vi "moveToTargetPosition.vi"(1 "speed":dbl=2000.0 min=0.0 max=2000.0, 2 "Encoder COM Port":refnum<visa-resource-name>, 3 "targetPos":dbl, 4 "currentPos":dbl) -> (0 "updatedCurrentPos":dbl)   [LabVIEW 2013]
panel:
  # "The default motor speed is 2000 steps/second."
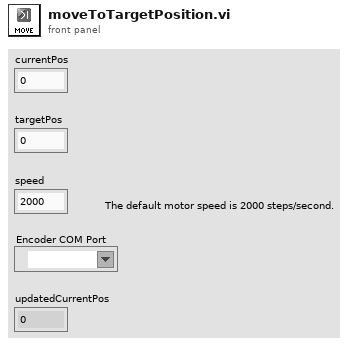
[diagram p1: front panel]
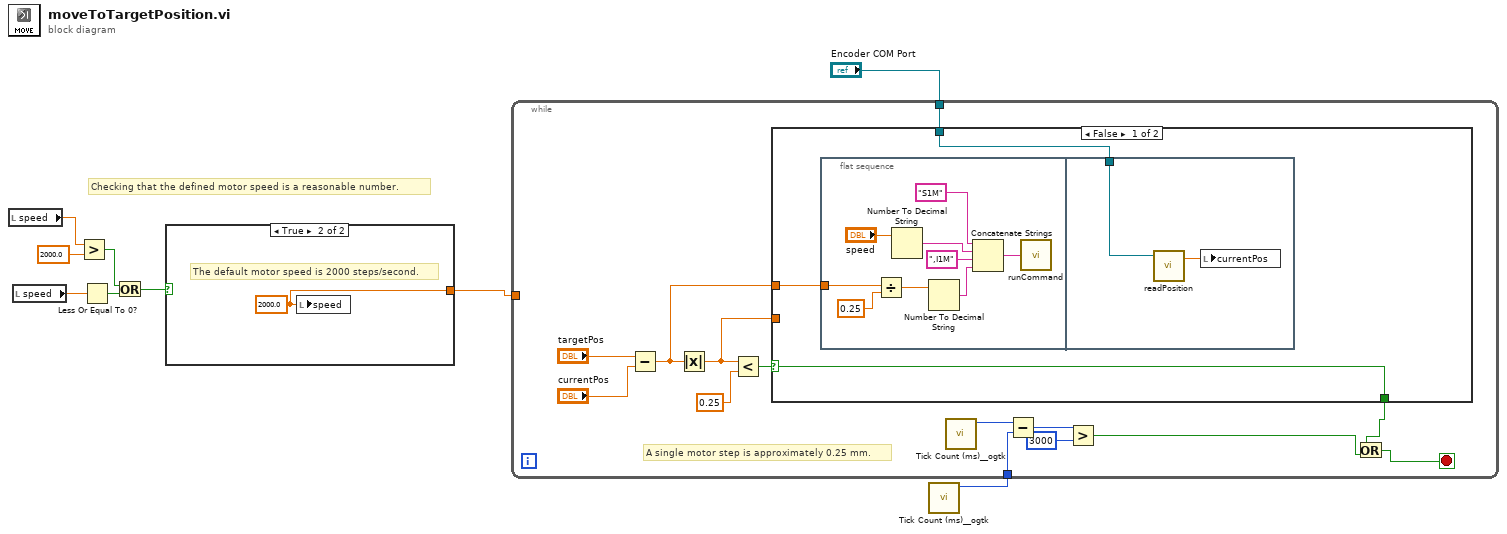
[diagram p0: block diagram]
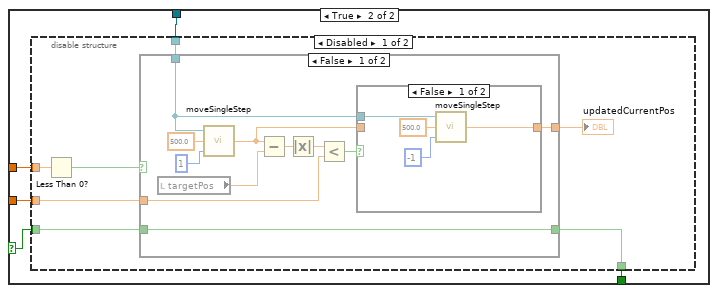
[diagram p3: hidden frame]
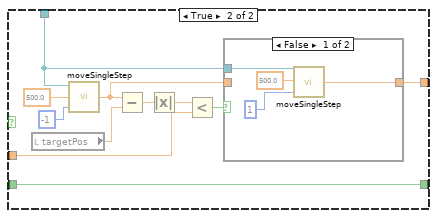
[diagram p5: hidden frame]
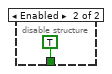
[diagram p7: hidden frame]
diagram:
  # "Checking that the defined motor speed is a reasonable number."
  n1 = local read "speed"() -> (w7:dbl)
  n2 = local read "speed"() -> (w4:dbl)
  n3 = Greater?(x=w7, y=2000.0) -> (0:w8:bool)
  n4 = Less Or Equal To 0?(x=w4) -> (x <= 0?=w6:bool)
  n5 = Or(x=w8, y=w6) -> (x .or. y?=w9:bool)
  n6 = case shown="True" w9 {
    tunnel: [_ w10] -> w2
    frame False {
    }
    frame True {
      w10 = 2000.0 ("speed")
      # "The default motor speed is 2000 steps/second."
      n7 = local write "speed"(w10) -> ()
    }
  }
  n8 = call <userlib>:"Tick Count (ms)__ogtk.vi"() -> ("millisecond timer value"=w1:u32)  [unwired: 10 in, 1 out]
  n9 = while {
    tunnel: "Encoder COM Port" -> [w18]
    tunnel: w2 -> [_]
    tunnel: w1 -> [w16]
    stop <- w11 stop-if-true
    # "A single motor step is approximately 0.25 mm."
    n10 = Subtract(x="targetPos", y="currentPos") -> (x-y=w21:dbl)
    n11 = Absolute Value(x=w21) -> (abs(x)=w19:dbl)
    n12 = Less?(x=w19, y=0.25) -> (x < y?=w22:bool)
    n13 = case shown="False" w22 {
      selector: w22 -> [w26 w41]
      tunnel: w21 -> [w27 w43]
      tunnel: w19 -> [_ w42]
      tunnel: [w26 w40] -> w12
      tunnel: w18 -> [w25 w39]
      frame False {
        n14 = flat-sequence {
          tunnel: w27 -> [w34]
          tunnel: w25 -> [w37]
          frame #0 {
            n15 = Divide(x=w34, y=0.25) -> (x/y=w32:dbl)
            n16 = Number To Decimal String(number="speed") -> (decimal integer string=w29:string)  [unwired: 1 in]
            n17 = Number To Decimal String(number=w32) -> (decimal integer string=w36:string)  [unwired: 1 in]
            n18 = Concatenate Strings("S1M" ("string"), w29, ",I1M" ("string"), w36) -> (w35:string)
            n19 = call "runCommand.vi"("command"=w35) -> ()  [unwired: 1 in]
          }
          frame #1 {
            n20 = call "readPosition.vi"("VISA resource name"=w37) -> ("position"=w38:dbl)  [unwired: 1 in, 2 out]
            n21 = local write "currentPos"(w38) -> ()
          }
        }
      }
      frame True {
        n22 = disable-structure shown="Disabled" {
          disable-tunnel: w43 -> [w50 _]
          disable-tunnel: w42 -> [w48 _]
          disable-tunnel: w41 -> [w47 _]
          disable-tunnel: [w46 TRUE] -> w40
          disable-tunnel: w39 -> [w44 _]
          frame Disabled {
            n23 = Less Than 0?(x=w50) -> (x < 0?=w49:bool)
            n24 = case shown="False" w49 {
              tunnel: w44 -> [w54 w71]
              tunnel: w48 -> [w55 w72]
              tunnel: w47 -> [w52 w68]
              tunnel: [w53 w69] -> w45
              tunnel: [w52 w68] -> w46
              frame False {
                n25 = local read "targetPos"() -> (w57:dbl)
                n26 = call "moveSingleStep.vi"("direction"=1, "motorSpeed"=500.0, "VISA resource name"=w54) -> ("position"=w61:dbl)
                n27 = Subtract(x=w61, y=w57) -> (x-y=w58:dbl)
                n28 = Absolute Value(x=w58) -> (abs(x)=w59:dbl)
                n29 = Less?(x=w59, y=w55) -> (x < y?=w60:bool)
                n30 = case shown="False" w60 {
                  tunnel: w61 -> [_ w66]
                  tunnel: w54 -> [w64 _]
                  tunnel: [w63 w66] -> w53
                  frame False {
                    n31 = call "moveSingleStep.vi"("direction"=-1, "motorSpeed"=500.0, "VISA resource name"=w64) -> ("position"=w63:dbl)
                  }
                  frame True {
                  }
                }
              }
              frame True {
                n32 = local read "targetPos"() -> (w76:dbl)
                n33 = call "moveSingleStep.vi"("direction"=-1, "motorSpeed"=500.0, "VISA resource name"=w71) -> ("position"=w70:dbl)
                n34 = Subtract(x=w70, y=w76) -> (x-y=w75:dbl)
                n35 = Absolute Value(x=w75) -> (abs(x)=w73:dbl)
                n36 = Less?(x=w73, y=w72) -> (x < y?=w74:bool)
                n37 = case shown="False" w74 {
                  tunnel: w71 -> [w81 _]
                  tunnel: w70 -> [_ w82]
                  tunnel: [w79 w82] -> w69
                  frame False {
                    n38 = call "moveSingleStep.vi"("direction"=1, "motorSpeed"=500.0, "VISA resource name"=w81) -> ("position"=w79:dbl)
                  }
                  frame True {
                  }
                }
              }
            }
            "updatedCurrentPos" <- w45
          }
          frame Enabled {
          }
        }
      }
    }
    n39 = call <userlib>:"Tick Count (ms)__ogtk.vi"() -> ("millisecond timer value"=w17:u32)  [unwired: 10 in, 1 out]
    n40 = Subtract(x=w17, y=w16) -> (x-y=w15:u32)
    n41 = Greater?(x=w15, y=u32 3000) -> (0:w13:bool)
    n42 = Or(x=w12, y=w13) -> (x .or. y?=w11:bool)
  }
